vi "USB_Error.vi"(11 "System Data":T1={"System"={"Active"=FALSE, "Exit"=FALSE, "Command wait"="", "Status_Time"=0, "Time_GPS"=0}, "Stepper Motor"={"Connection Reference"="", "Valid Connection"=FALSE, "Speed"=15}, "Camera Data"={"Image path"=path "", "Filenames"=[], "Filenames queue"=[]}, "Core"={"Close Panel on Exit?"=FALSE, "Current VI Reference"=refnum}} {"Stepper Motor"."Speed" scale=0.0..30.0}) -> (0 "Connection":bool, 3 "System Data out":T1={"System"={"Active"=FALSE, "Exit"=FALSE, "Command wait"="", "Status_Time"=0, "Time_GPS"=0}, "Stepper Motor"={"Connection Reference"="", "Valid Connection"=FALSE, "Speed"=15}, "Camera Data"={"Image path"=path "", "Filenames"=[], "Filenames queue"=[]}, "Core"={"Close Panel on Exit?"=FALSE, "Current VI Reference"=refnum}} {"Stepper Motor"."Speed" scale=0.0..30.0})   [LabVIEW 2019]
uses:
  System Data.ctl
  Stepper Data.ctl
  Camera Data.ctl
  002519a6-9b4b-4608-a0a2-f5652379bb88.vi
  <extravilib>/ChannelInstances/Tag-bool/Read With Abort.vi
  <extravilib>/ChannelInstances/Tag-bool/Write With Abort.vi
  <extravilib>/ChannelInstances/Tag-bool/Instantiate.vi
  <extravilib>/ChannelInstances/Tag-bool/Endpoint.vi
  <extravilib>/ChannelInstances/Tag-bool/EndpointRead.vi
  <extravilib>/ChannelInstances/Tag-bool.lvlib
panel:
  out "Pict Ring 2":dbl(ring)
  out "String":string="System Connection Error!\nCheck USB connection"
  out "Pict Ring":dbl(ring)=2.0
  in  "Stop":bool
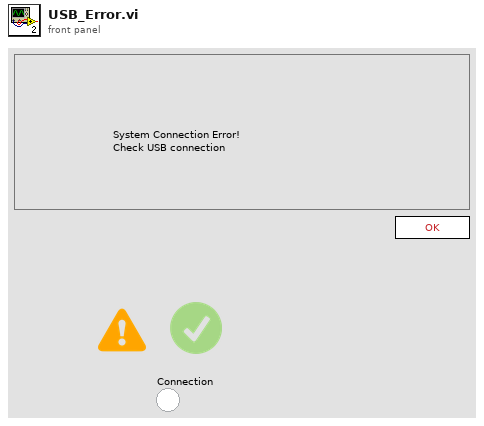
[diagram p1: front panel]
types:
  T1 = typedef "System Data.ctl" = cluster{"System":cluster{"Active":bool, "Exit":bool, "Command wait":string, "Status_Time":i32, "Time_GPS":i32}, "Stepper Motor":T2, "Camera Data":T3, "Core":cluster{"Close Panel on Exit?":bool, "Current VI Reference":refnum<vi>}}
  T2 = typedef "Stepper Data.ctl" = cluster{"Connection Reference":refnum<visa-resource-name>, "Valid Connection":bool, "Speed":i32}
  T3 = typedef "Camera Data.ctl" = cluster{"Image path":path, "Filenames":string[], "Filenames queue":string[]}
  T4 = typedef "Tag-bool.lvlib/))Channel.ctl" = refnum<queue>
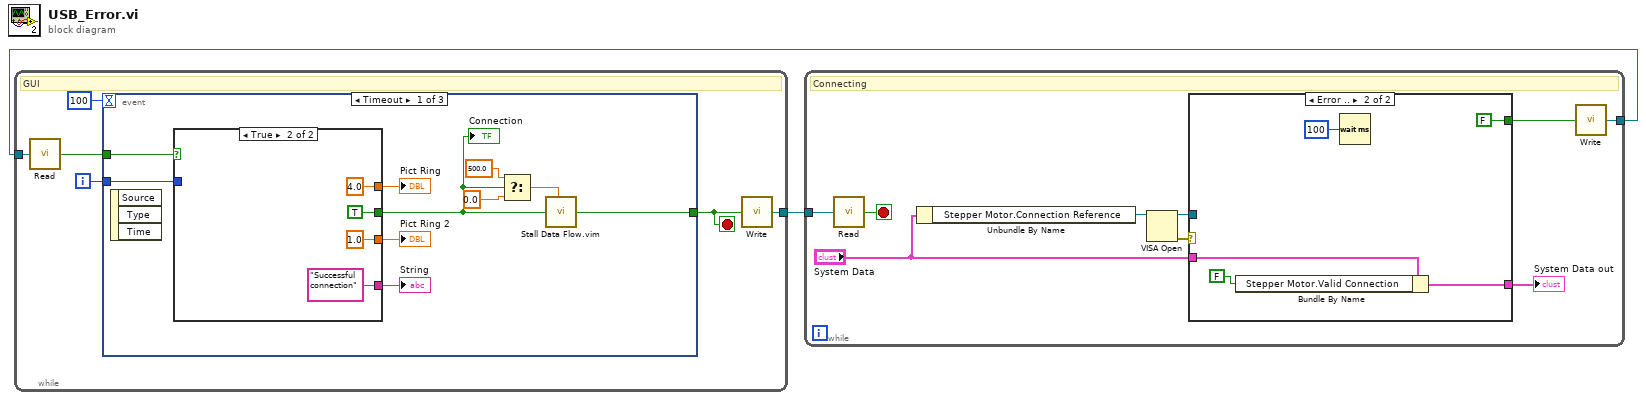
[diagram p0: block diagram]
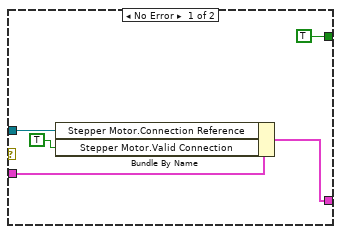
[diagram p2: hidden frame]
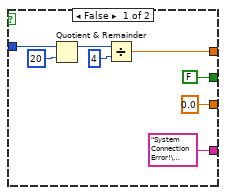
[diagram p3: hidden frame]
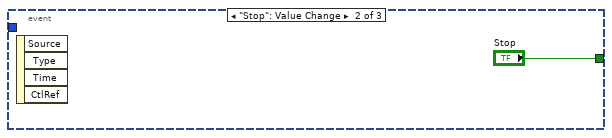
[diagram p4: hidden frame]
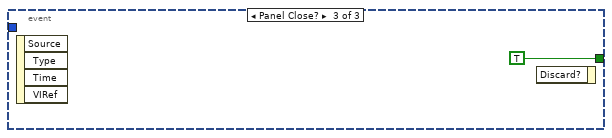
[diagram p5: hidden frame]
diagram:
  n1 = while {
    tunnel: [w5] -> w2
    tunnel: w1 -> [w4]
    i -> [w7]
    stop <- w6 stop-if-true
    # "GUI"
    n2 = call <extravilib>:"Read.vi"("channel"=w4) -> ("element"=w3:bool)  [unwired: 1 in, 1 out]
    n3 = event shown="[0] Timeout" {
      selector: _ -> [_ _ _]
      dyn-events: _ -> [_ _ _]
      timeout: u32 100 ("milliseconds to wait") -> [_ _ _]
      tunnel: w7 -> [w16 _ _]
      tunnel: [w9 "Stop" TRUE ("Stop")] -> w6
      tunnel: w3 -> [w14 _ _]
      event Timeout {
        n4 = event-data() -> ()  [unwired: 1 in, 3 out]
        n5 = case shown="True" w14 {
          tunnel: [0.0 ("Pict Ring 2") 1.0 ("Pict Ring 2")] -> w17
          tunnel: ["System Connection Error!\nCheck USB connection" ("String") "Successful connection" ("String")] -> w18
          tunnel: w16 -> [w21 _]
          tunnel: [w20 4.0] -> w15
          tunnel: [FALSE TRUE] -> w13
          frame False {
            n6 = Quotient & Remainder(x=w21, y=20) -> (x-y*floor(x/y)=w24:i32)  [unwired: 1 out]
            n7 = Divide(x=w24, y=4 ("x")) -> (x/y=w20:dbl)
          }
          frame True {
          }
        }
        "Pict Ring" <- w15
        "Pict Ring 2" <- w17
        "String" <- w18
        "Connection" <- w13
        n8 = Select(t=500.0, s=w13, f=0.0) -> (s? t:f=w12:dbl)
        n9 = call "Stall Data Flow.vim"("value in"=w13, "milliseconds to wait"=w12) -> ("value out"=w9:bool)  [unwired: 1 out]
      }
      event "Stop": Value Change {
        n10 = event-data() -> ()  [unwired: 1 in, 4 out]
      }
      event Panel Close? {
        n11 = event-data() -> ()  [unwired: 1 in, 4 out]
        n12 = event-data() -> ()  [unwired: 2 in, 1 out]
      }
    }
    n13 = call <extravilib>:"Write.vi"("element"=w6) -> ("channel"=w5:T4)  [unwired: 1 out]
  }
  n14 = while {
    tunnel: w2 -> [w41]
    tunnel: [w39] -> w1
    stop <- w40 stop-if-true
    # "Connecting"
    n15 = call <extravilib>:"Read.vi"("channel"=w41) -> ("element"=w40:bool)  [unwired: 1 in, 1 out]
    n16 = Unbundle By Name("System Data") -> ("Stepper Motor.Connection Reference"=w38:refnum<visa-resource-name>)
    n17 = VISA Open(VISA resource name=w38) -> (VISA resource name=w35:refnum<visa-resource-name>, error out=w37:errorcluster)  [unwired: 4 in]
    n18 = case shown="Error .." w37 {
      tunnel: [TRUE FALSE] -> w36
      tunnel: "System Data" -> [w45 w49]
      tunnel: w35 -> [w44 _]
      tunnel: [w42 w48] -> w34
      frame No Error {
        n19 = Bundle By Name(cluster=w45, "Stepper Motor.Connection Reference"=w44, "Stepper Motor.Valid Connection"=TRUE) -> (w42:T1)
      }
      frame Error {
        n20 = Bundle By Name(cluster=w49, "Stepper Motor.Valid Connection"=FALSE) -> (w48:T1)
        n21 = Wait (ms)(milliseconds to wait=u32 100) -> ()  [unwired: 1 out]
      }
    }
    "System Data out" <- w34
    n22 = call <extravilib>:"Write.vi"("element"=w36) -> ("channel"=w39:T4)  [unwired: 1 out]
  }
